vi "Start Haptic Loop.vi"(8 "error in (no error)":errorcluster, 10 "Mode Selection":u16(ring) items=["Custom Mode", "Read Mode", "Write Mode"]) -> (0 "error out":errorcluster)   [LabVIEW 2021, in "Haptic Prog Interface.lvlib"]
doc: "Begins the haptic loop, must be ran before any other VI from the library is ran."
uses:
  Haptic Prog Interface.lvlib
  Haptic-Programming-Interface/src/x64/Debug/Haptic Programming Interface.dll
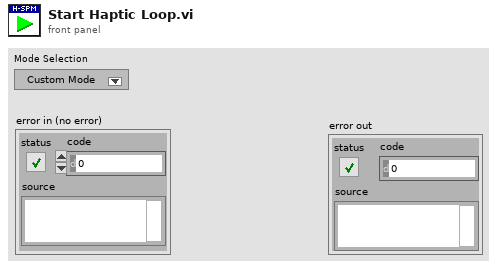
[diagram p1: front panel]
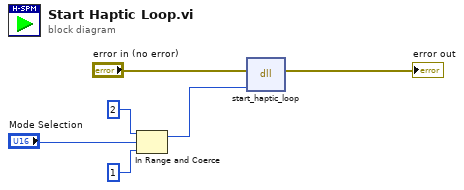
[diagram p0: block diagram]
diagram:
  n1 = In Range and Coerce(upper limit=2, x="Mode Selection", lower limit=1) -> (coerced(x)=w2:i32)  [unwired: 1 out]
  n2 = dll-call lib="C:/Users/freem/Documents/GitHub/Haptic-Programming-Interface/src/x64/Debug/Haptic Programming Interface.dll" fn="start_haptic_loop"(error in="error in (no error)", "input"=w2) -> (error out=→"error out":errorcluster)  [unwired: 4 in, 1 out]
